vi "Start.vi"(11 "Custom Device in":refnum<class "Custom Device.lvclass">) -> (0 "error out":errorcluster, 3 "Custom Device out":refnum<class "Custom Device.lvclass">)   [LabVIEW 2027, in "Custom Device Interfaces.lvlib" / "Custom Device.lvclass"]
uses:
  Custom Device.lvclass
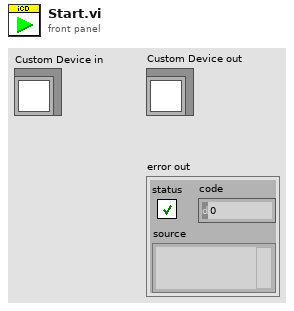
[diagram p1: front panel]
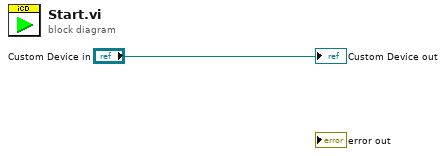
[diagram p0: block diagram]
diagram:
  "Custom Device out" <- "Custom Device in"
